vi "Muxed_Acquisition_withDC.vi"() -> ()   [LabVIEW 2018]
uses:
  <vilib>/rvi/Emulation/niFpgaGetClockAttributes.vi
  <vilib>/rvi/Emulation/niFpgaSctlEmulationGetInTimedLoop.vi
  <vilib>/rvi/Emulation/niFpgaEmulationReportErrorSimple.vi
  <vilib>/rvi/eio/common/nirviEmuTemplateMethod_errors.vi
  <vilib>/rvi/interface/RandomDataEmulation/niFpgaRandomDataHandleErrors.vi
  <vilib>/rvi/Emulation/niFpgaCriticalErrorInLSC.vi
  <vilib>/eio/EIONode/EIONode.xnode
  <vilib>/rvi/DataTransferAndStorage/Container/XNode/niFpgaContainer.xnode
  <vilib>/rvi/interface/RandomDataEmulation/nirviRandomDataFpgaReadWriteTemplate.vi
panel:
  out "DC component":i16
  out "DC FIFO":bool
  out "DC acquisition":bool
  in  "DC-Sampling":u32 caption="Count(Ticks)"
  out "Read Value":i16
  out "FIFO timeout":bool
  in  "Numeric":i16
  in  "Sampling(Ticks)":u32 caption="Count(Ticks)"
  out "Acquisition\nTimeout":bool
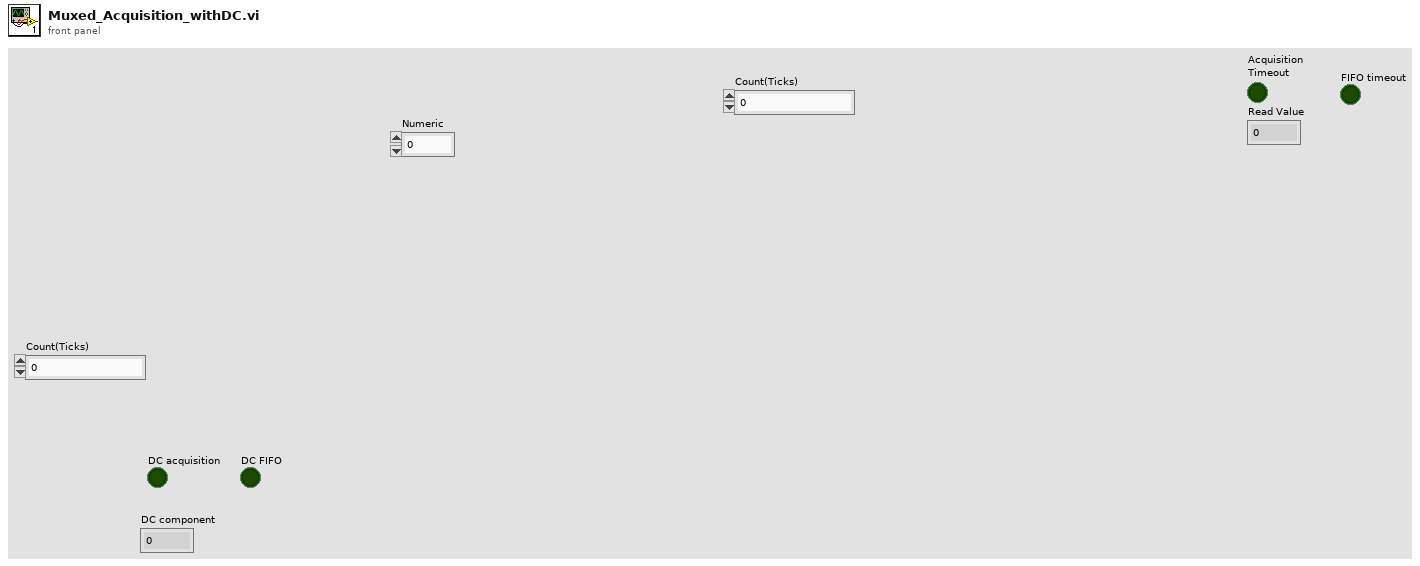
[diagram p1: front panel]
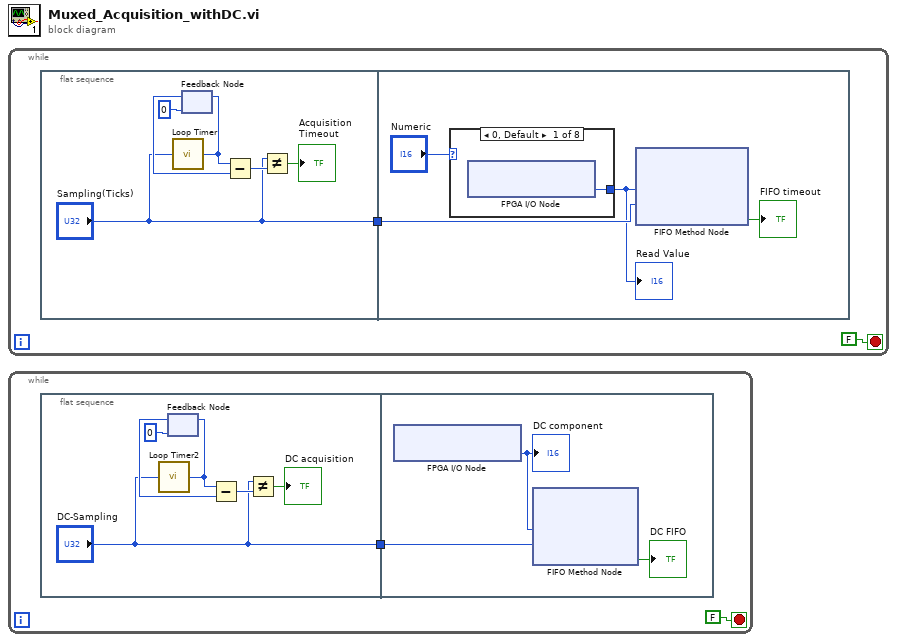
[diagram p0: block diagram]
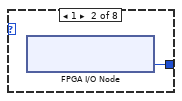
[diagram p2: hidden frame]
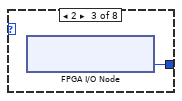
[diagram p3: hidden frame]
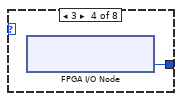
[diagram p4: hidden frame]
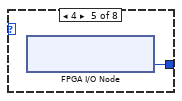
[diagram p5: hidden frame]
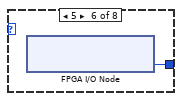
[diagram p6: hidden frame]
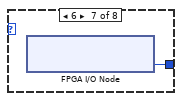
[diagram p7: hidden frame]
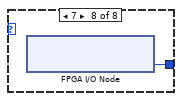
[diagram p8: hidden frame]
diagram:
  n1 = while {
    stop <- FALSE stop-if-true
    n2 = flat-sequence {
      tunnel: ["Sampling(Ticks)"] -> w1
      tunnel: w1 -> [w12]
      frame #0 {
        n3 = call "Loop Timer"("Count(Ticks)"="Sampling(Ticks)") -> ("Tick Count(Ticks)"=w7:u32)
        n4 = feedback-in #1(w7) -> ()
        n5 = feedback #1(u32 0 ("Tick Count(Ticks)")) -> (w6:u32)
        n6 = Subtract(x=w7, y=w6) -> (x-y=w5:u32)
        n7 = Not Equal?(x="Sampling(Ticks)", y=w5) -> (x != y?=→"Acquisition\nTimeout":bool)
      }
      frame #1 {
        n8 = case shown="0, Default" "Numeric" {
          tunnel: [w13 w14 w15 w16 w17 w18 w19 w20] -> w10
          frame 0, Default {
            n9 = xnode "FPGA I/O Node"() -> ("Connector0/AI0"=w13:i16)  [unwired: 1 in, 1 out]
          }
          frame 1 {
            n10 = xnode "FPGA I/O Node"() -> ("Connector0/AI1"=w14:i16)  [unwired: 1 in, 1 out]
          }
          frame 2 {
            n11 = xnode "FPGA I/O Node"() -> ("Connector0/AI2"=w15:i16)  [unwired: 1 in, 1 out]
          }
          frame 3 {
            n12 = xnode "FPGA I/O Node"() -> ("Connector0/AI3"=w16:i16)  [unwired: 1 in, 1 out]
          }
          frame 4 {
            n13 = xnode "FPGA I/O Node"() -> ("Connector0/AI4"=w17:i16)  [unwired: 1 in, 1 out]
          }
          frame 5 {
            n14 = xnode "FPGA I/O Node"() -> ("Connector0/AI5"=w18:i16)  [unwired: 1 in, 1 out]
          }
          frame 6 {
            n15 = xnode "FPGA I/O Node"() -> ("Connector0/AI6"=w19:i16)  [unwired: 1 in, 1 out]
          }
          frame 7 {
            n16 = xnode "FPGA I/O Node"() -> ("Connector0/AI7"=w20:i16)  [unwired: 1 in, 1 out]
          }
        }
        "Read Value" <- w10
        n17 = xnode ("FIFO Method Node")("Element"=w10, "Timeout"=w12) -> ("Timed Out?"=→"FIFO timeout":bool)  [unwired: 1 in, 1 out]
      }
    }
  }
  n18 = while {
    stop <- FALSE stop-if-true
    n19 = flat-sequence {
      tunnel: ["DC-Sampling"] -> w21
      tunnel: w21 -> [w30]
      frame #0 {
        n20 = call "Loop Timer2"("Count(Ticks)"="DC-Sampling") -> ("Tick Count(Ticks)"=w27:u32)
        n21 = feedback-in #2(w27) -> ()
        n22 = feedback #2(u32 0 ("Tick Count(Ticks)")) -> (w26:u32)
        n23 = Subtract(x=w27, y=w26) -> (x-y=w25:u32)
        n24 = Not Equal?(x="DC-Sampling", y=w25) -> (x != y?=→"DC acquisition":bool)
      }
      frame #1 {
        n25 = xnode "FPGA I/O Node"() -> ("Connector0/AI7"=w31:i16)  [unwired: 1 in, 1 out]
        "DC component" <- w31
        n26 = xnode ("FIFO Method Node")("Element"=w31, "Timeout"=w30) -> ("Timed Out?"=→"DC FIFO":bool)  [unwired: 1 in, 1 out]
      }
    }
  }
